vi "Get Hardware Relay State.vi"(0 "PhysicalChannelRelay in":refnum<class "PhysicalChannelRelay.lvclass">, 5 "Session Handle in":T1, 11 "error in (no error)":errorcluster) -> (4 "PhysicalChannelRelay out":refnum<class "PhysicalChannelRelay.lvclass">, 10 "RelayPosition":T2=10 caption="position" items=["Open"=10, "Closed"=11], 15 "error out":errorcluster)   [LabVIEW 2015, in "SLSC Switch.lvlib" / "PhysicalChannelRelay.lvclass"]
doc: "This uses a phyiscal channel to get the current hardware state of a relay."
uses:
  PhysicalChannelRelay.lvclass
  slscsl/RelayPosition.ctl
  SLSC Session/Typedefs/Session Handle.ctl
  SLSC Session/SLSC Session.lvclass
  PhysicalChannelRelay.lvclass/PhysicalChannelRelay.ctl
  slscsl/slscsl.lvclass
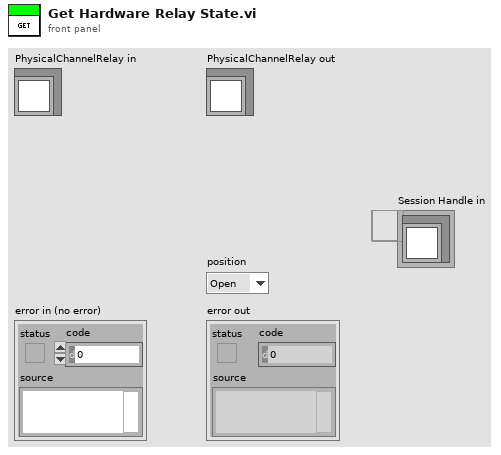
[diagram p1: front panel]
types:
  T1 = typedef "SLSC Switch.lvlib/SLSC Session.lvclass/Session Handle.ctl" = refnum<data-value>
  T2 = typedef "SLSC Switch.lvlib/slscsl.lvclass/RelayPosition.ctl" = i32
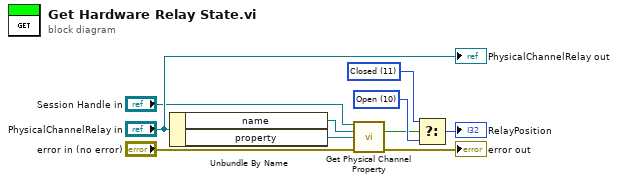
[diagram p0: block diagram]
diagram:
  w8 = T2 10 items=["Open"=10, "Closed"=11] ("f")
  w9 = T2 11 items=["Open"=10, "Closed"=11] ("RelayPosition")
  n1 = Unbundle By Name("PhysicalChannelRelay in") -> ("name"=w5:refnum<k21>, "property"=w4:refnum<k21>)
  n2 = call "Get Physical Channel Property.vi"("Session Handle in"="Session Handle in", "physical channel"=w5, "property"=w4, "error in (no error)"="error in (no error)") -> ("property value"=w3:bool, "error out"=→"error out":errorcluster)  [unwired: 9 in, 1 out]
  n3 = Select(t=w9, s=w3, f=w8) -> (s? t:f=→"RelayPosition":T2)
  "PhysicalChannelRelay out" <- "PhysicalChannelRelay in"
